vi "TriggerPressed.vi"(11 "Trigger Value":dbl) -> (3 "Pressed?":bool)   [LabVIEW 2020]
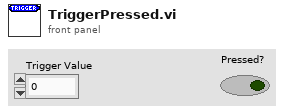
[diagram p1: front panel]
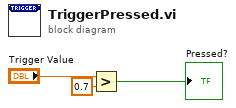
[diagram p0: block diagram]
diagram:
  n1 = Greater?(x="Trigger Value", y=0.7) -> (0:→"Pressed?":bool)
